vi "demo.vi"() -> ()   [LabVIEW 2012]
uses:
  <vilib>/Utility/miscctls.llb/LVPositionTypeDef.ctl
  SubVIs/typedef/User_Data_Cluster.ctl
  SubVIs/typedef/User Accounts.ctl
  type def/nodos.ctl
  type def/Hyde&Show.ctl
panel:
  out "INT \nRead":u16[](array[numeric])
  out "REAL \nRead":sgl[](array[numeric])
  out "BOOL \nRead":bool
  out "Cluster":T1
  in  "Video 2":bool
  in  "User-data cluster":T2
  out "Position":T4
  out "WS":picture
  out "Box":picture
  out "?":errorcluster
  in  "Admin Options":u16(ring)=1 items=["None", "1/ New User", "2/ Read&Modify Users", "3/ Read Log"]
  in  "Video":bool
  in  "?":bool
  in  "?":T5(tab)
  out "back ground":picture
  in  "error in (no error)":errorcluster
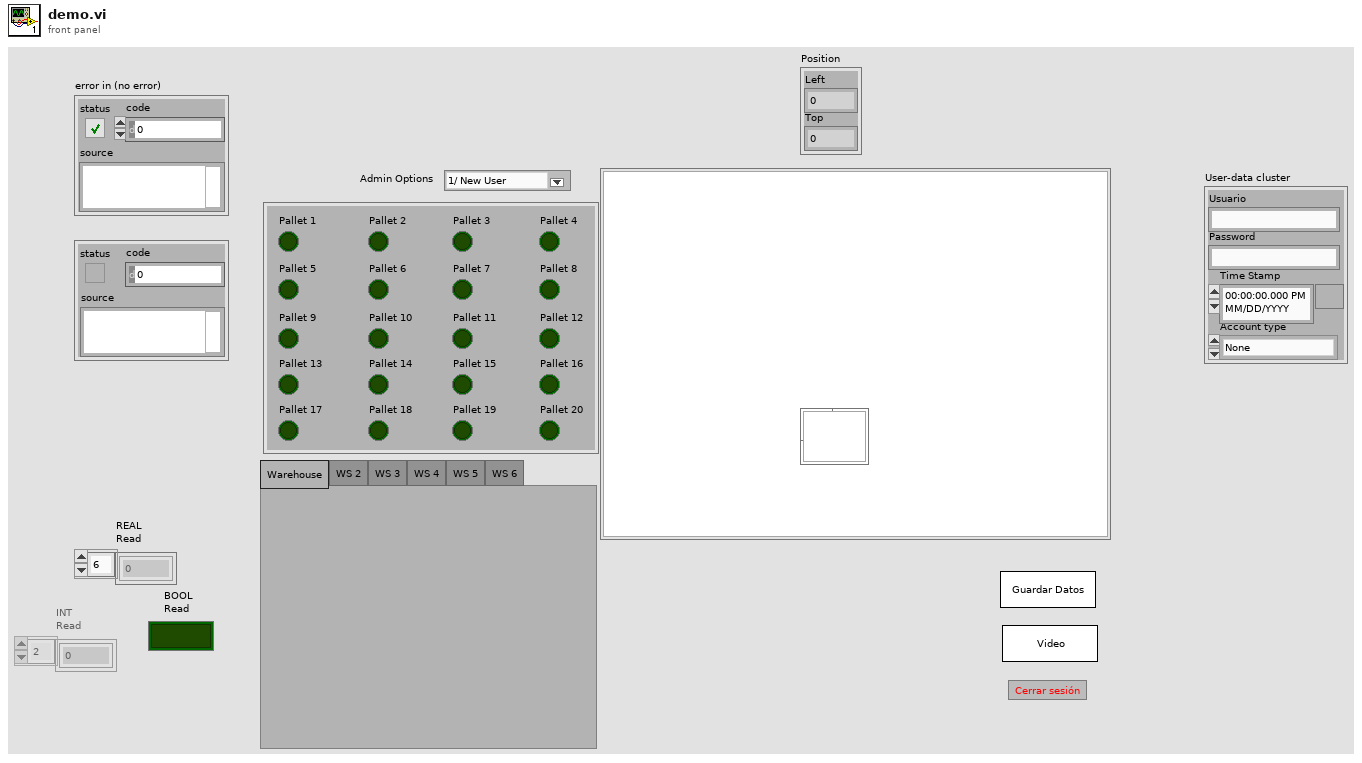
[diagram p1: front panel]
types:
  T1 = cluster{"Pallet 1":bool, "Pallet 2":bool, "Pallet 3":bool, "Pallet 4":bool, "Pallet 5":bool, "Pallet 6":bool, "Pallet 7":bool, "Pallet 8":bool, "Pallet 9":bool, "Pallet 10":bool, "Pallet 11":bool, "Pallet 12":bool, "Pallet 13":bool, "Pallet 14":bool, "Pallet 15":bool, "Pallet 16":bool, "Pallet 17":bool, "Pallet 18":bool, "Pallet 19":bool, "Pallet 20":bool}
  T2 = typedef "User_Data_Cluster.ctl" = cluster{"Usuario":string, "Password":string, "Account type":T3, "Time Stamp":timestamp}
  T3 = typedef "User Accounts.ctl" = enum16{"None", "User", "Admin"}
  T4 = typedef "LVPositionTypeDef.ctl" = cluster{"Left":i32, "Top":i32}
  T5 = enum32{"Warehouse", "WS 2", "WS 3", "WS 4", "WS 5", "WS 6"}
  T6 = cluster{"TCP Connection":refnum<k5>, "Session":u8[], "EtherNet/IP Device Address":string}
  T7 = typedef "nodos.ctl" = enum16{"Default", "Login", "Create", "Running", "Cluse User", "Close Conections", "End"}
  T8 = typedef "Hyde&Show.ctl" = enum8{"Enabled", "Disabled", "Disabled and Grayed Out", "Hide"}
  T9 = typedef "imagedata.ctl" = cluster{"image type":i32, "image depth":i32, "image":u8[], "mask":u8[], "colors":u32[], "Rectangle":cluster{"left":i16, "top":i16, "right":i16, "bottom":i16}}
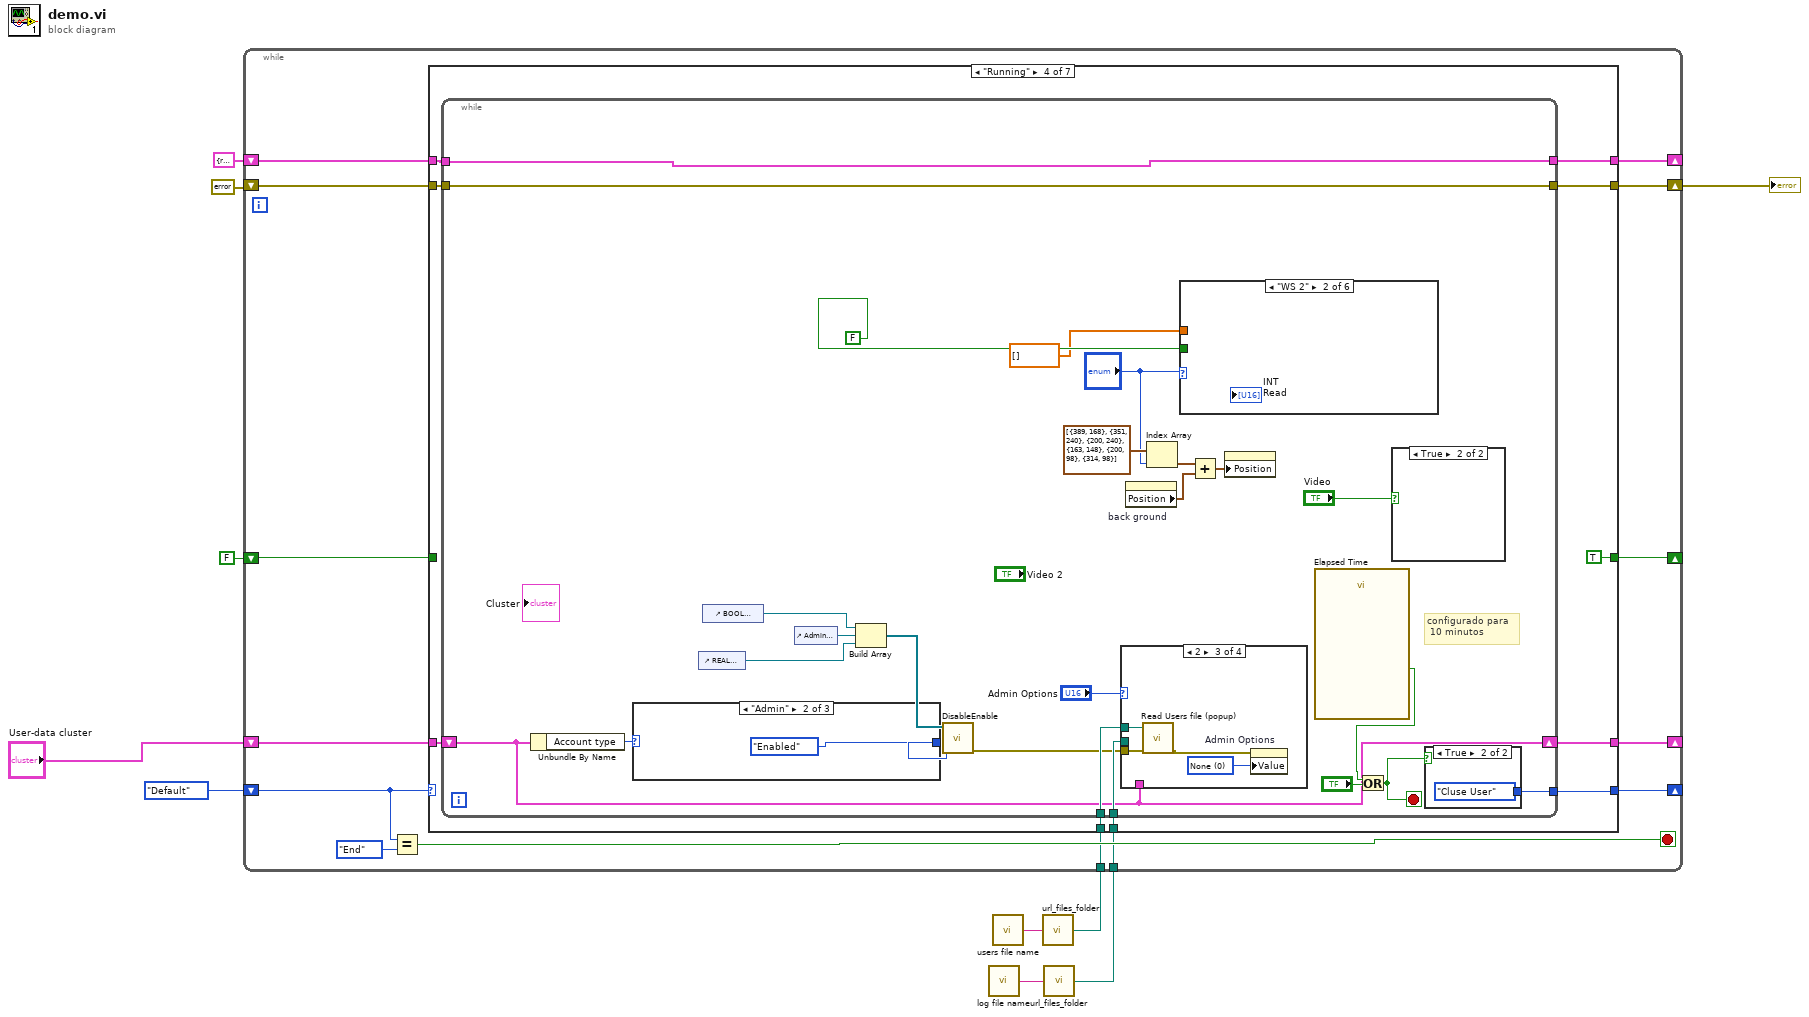
[diagram p0: block diagram]
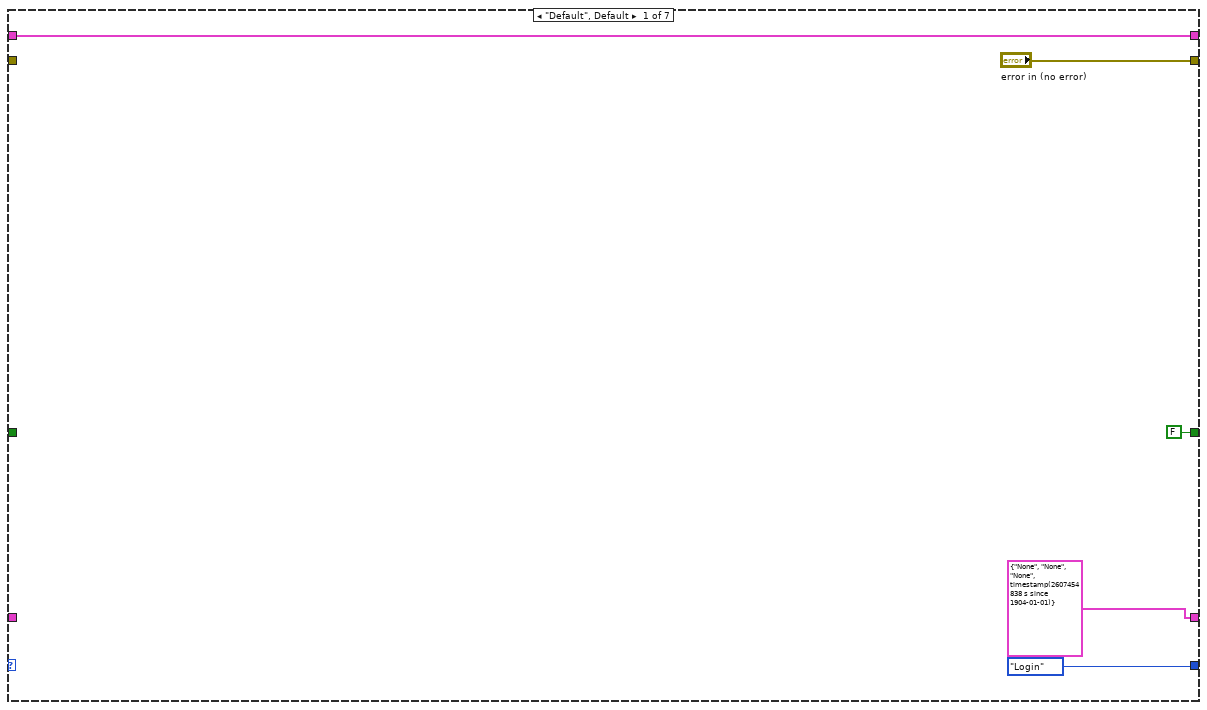
[diagram p2: hidden frame]
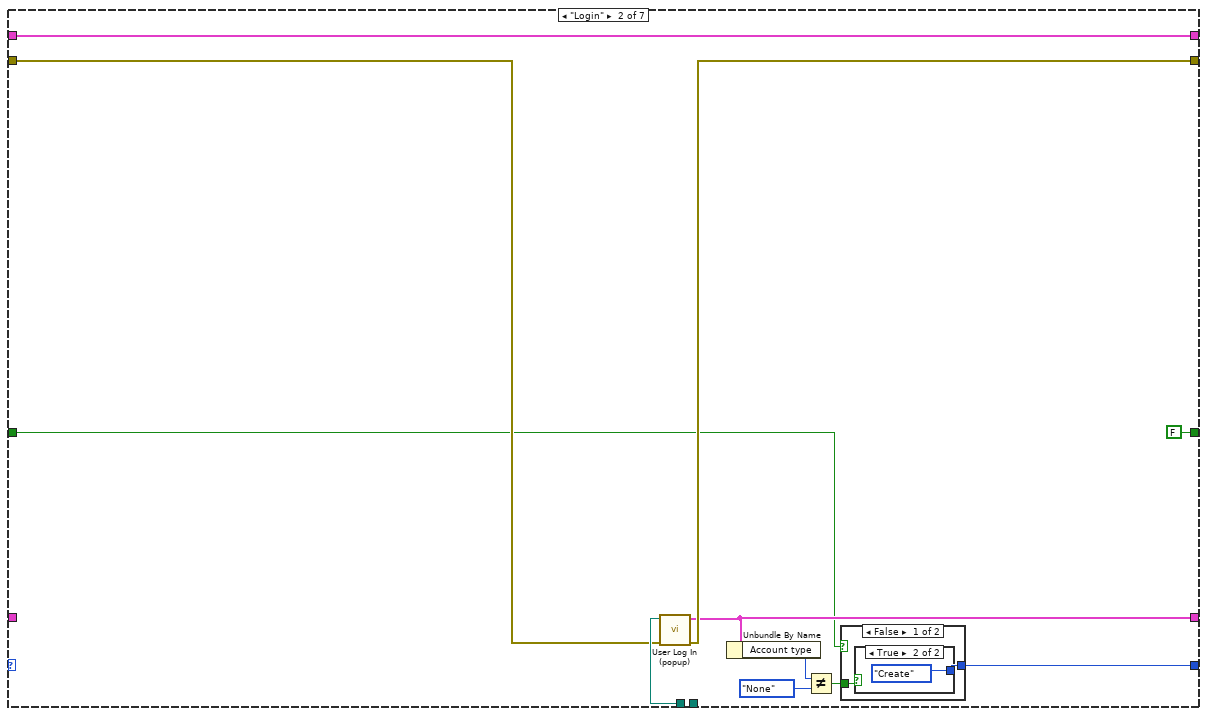
[diagram p3: hidden frame]
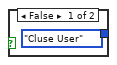
[diagram p4: hidden frame]
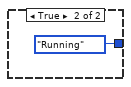
[diagram p5: hidden frame]
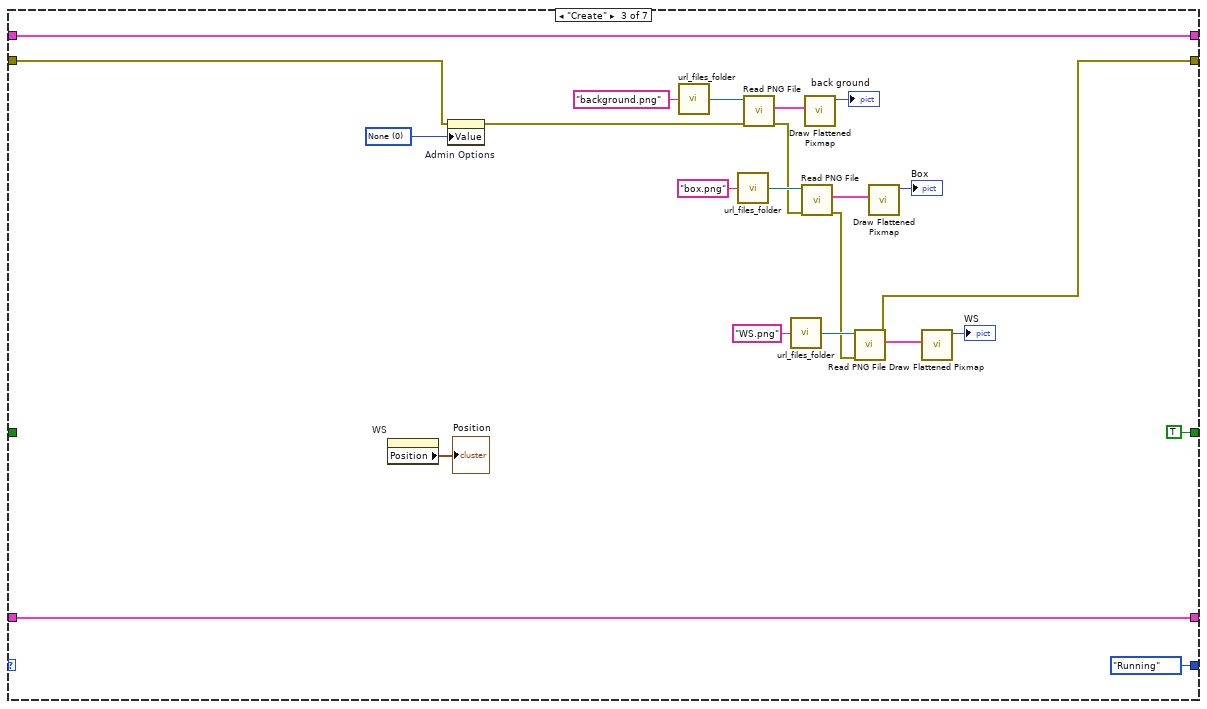
[diagram p6: hidden frame]
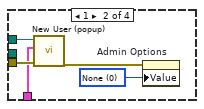
[diagram p8: hidden frame]
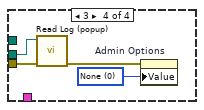
[diagram p9: hidden frame]
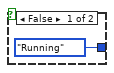
[diagram p10: hidden frame]
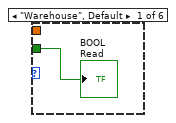
[diagram p12: hidden frame]
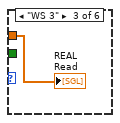
[diagram p13: hidden frame]
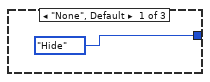
[diagram p17: hidden frame]
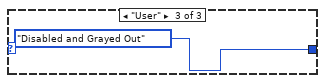
[diagram p18: hidden frame]
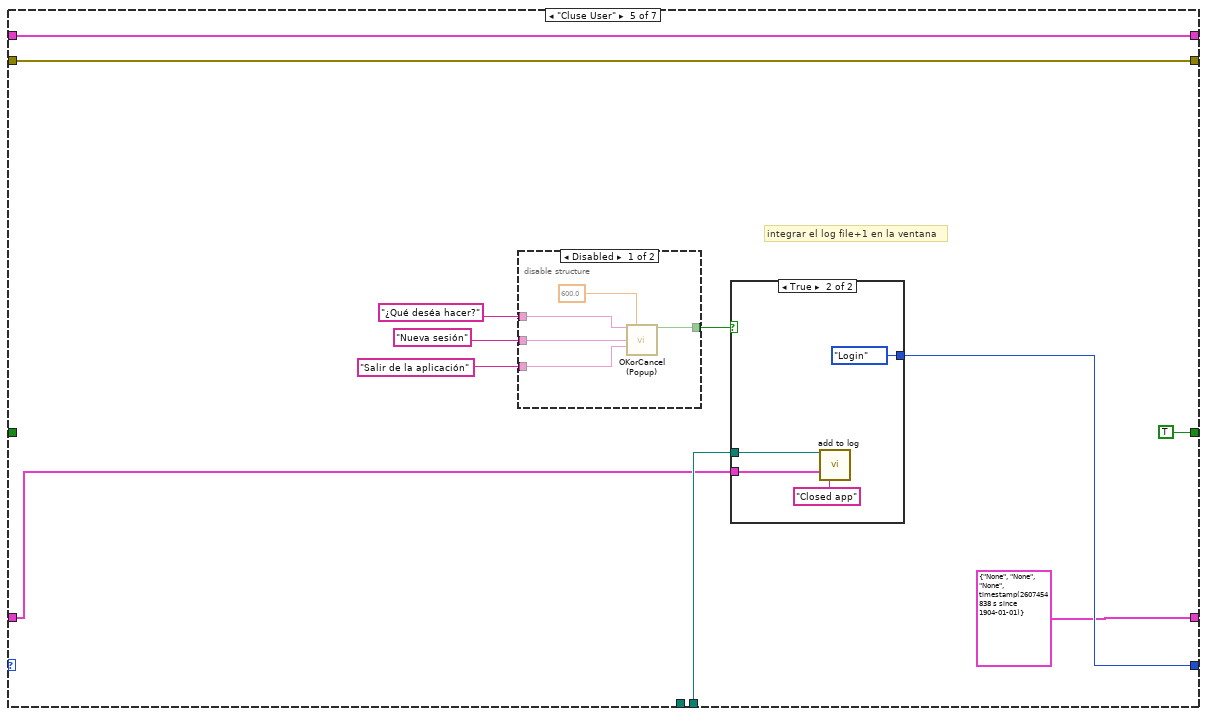
[diagram p19: hidden frame]
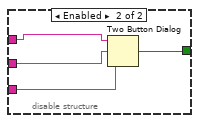
[diagram p20: hidden frame]
diagram:
  n1 = call "log file name.vi"() -> ("file name"=w4:string)  [unwired: 15 in]
  n2 = call "users file name.vi"() -> ("file name"=w6:string)  [unwired: 15 in]
  n3 = call "url_files_folder.vi"("file name"=w6) -> ("Path"=w5:path)  [unwired: 14 in]
  n4 = call "url_files_folder.vi"("file name"=w4) -> ("Path"=w3:path)  [unwired: 14 in]
  n5 = while {
    shift-right: [w23] -> _
    shift-left: nodos."Default" -> [w24]
    shift-right: [w16] -> w7
    shift-left: errorcluster {"status"=FALSE, "code"=0, "source"=""} ("error out") -> [w22]
    shift-right: [w19] -> _
    shift-left: "User-data cluster" -> [w17]
    shift-right: [w15] -> _
    shift-left: T6 {"TCP Connection"=refnum, "Session"=[], "EtherNet/IP Device Address"=""} ("Connection Cluster") -> [w18]
    tunnel: w5 -> [w14]
    tunnel: w3 -> [w13]
    shift-right: [w12] -> _
    shift-left: FALSE -> [w11]
    stop <- w20 stop-if-true
    n6 = Equal?(x=w24, y=nodos."End") -> (x = y?=w20:bool)
    n7 = case shown="\"Running\"" w24 {
      tunnel: [nodos."Login" w38 nodos."Running" w70 w134 nodos."End" nodos."End"] -> w23
      tunnel: ["error in (no error)" w34 w50 w75 w124 w149 w156] -> w16
      tunnel: w22 -> [_ w35 w47 w78 w124 w149 w156]
      tunnel: [T2 {"Usuario"="None", "Password"="None", "Account type"=enum."None", "Time Stamp"=timestamp(2607454838.413 s since 1904-01-01)} ("User-data cluster 2") w32 w64 w71 T2 {"Usuario"="None", "Password"="None", "Account type"=enum."None", "Time Stamp"=timestamp(2607454838.413 s since 1904-01-01)} ("User-data cluster 2") w152 T2 {"Usuario"="None", "Password"="None", "Account type"=enum."None", "Time Stamp"=timestamp(2607454838.413 s since 1904-01-01)} ("User-data cluster 2")] -> w19
      tunnel: w18 -> [w27 w36 w46 w77 w125 w150 w157]
      tunnel: w17 -> [_ _ w64 w74 w131 w152 _]
      tunnel: [w27 w36 w46 w76 w125 w150 w157] -> w15
      tunnel: w14 -> [_ w37 _ w72 _ _ _]
      tunnel: w13 -> [_ _ _ w73 w133 _ _]
      tunnel: [FALSE FALSE TRUE TRUE TRUE FALSE FALSE] -> w12
      tunnel: w11 -> [_ w30 _ _ _ _ _]
      frame "Default", Default {
      }
      frame "Login" {
        n8 = call "User Log In (popup).vi"("error in (no error)"=w35, 11:w37) -> ("error out"=w34:errorcluster, "User-data cluster Out"=w32:T2)  [unwired: 8 in]
        n9 = Unbundle By Name(w32) -> ("Account type"=w33:T3)
        n10 = Not Equal?(x=w33, y=User_Accounts."None") -> (x != y?=w40:bool)
        n11 = case shown="False" w30 {
          tunnel: w40 -> [w42 _]
          tunnel: [w41 nodos."Running"] -> w38
          frame False {
            n12 = case shown="True" w42 {
              tunnel: [nodos."Cluse User" nodos."Create"] -> w41
              frame False {
              }
              frame True {
              }
            }
          }
          frame True {
          }
        }
      }
      frame "Create" {
        w65 = u16 0 items=["None", "1/ View Users", "2/ Read Log", "3/ Modify Users", "4/ New User"] ("Admin Options")
        n13 = property on="WS" class="Pict"() -> ("Position"=→"Position":T4)  [unwired: 2 in, 2 out]
        n14 = property on="Admin Options" class="Ring (strict)"(error in=w47, "Value"=w65) -> (error out=w58:errorcluster)  [unwired: 1 in, 1 out]
        n15 = call "url_files_folder.vi"("file name"="background.png") -> ("Path"=w59:path)  [unwired: 14 in]
        n16 = call "url_files_folder.vi"("file name"="box.png") -> ("Path"=w60:path)  [unwired: 14 in]
        n17 = call <vilib>:"Read PNG File.vi"("error in (no error)"=w58, "path to PNG file"=w59) -> ("error out"=w57:errorcluster, "image data"=w68:T9)  [unwired: 7 in, 1 out]
        n18 = call "url_files_folder.vi"("file name"="WS.png") -> ("Path"=w53:path)  [unwired: 14 in]
        n19 = call <vilib>:"Read PNG File.vi"("error in (no error)"=w57, "path to PNG file"=w60) -> ("error out"=w51:errorcluster, "image data"=w66:T9)  [unwired: 7 in, 1 out]
        n20 = call <vilib>:"Draw Flattened Pixmap.vi"("image data"=w68) -> ("new picture"=→"back ground":picture)  [unwired: 8 in]
        n21 = call <vilib>:"Read PNG File.vi"("error in (no error)"=w51, "path to PNG file"=w53) -> ("error out"=w50:errorcluster, "image data"=w55:T9)  [unwired: 7 in, 1 out]
        n22 = call <vilib>:"Draw Flattened Pixmap.vi"("image data"=w66) -> ("new picture"=→"Box":picture)  [unwired: 8 in]
        n23 = call <vilib>:"Draw Flattened Pixmap.vi"("image data"=w55) -> ("new picture"=→"WS":picture)  [unwired: 8 in]
      }
      frame "Running" {
        n24 = while {
          tunnel: w78 -> [w81]
          tunnel: w77 -> [w82]
          tunnel: [w82] -> w76
          tunnel: [w81] -> w75
          shift-right: [w84] -> w71
          shift-left: w74 -> [w84]
          tunnel: w73 -> [w95]
          tunnel: w72 -> [w91]
          tunnel: [w94] -> w70
          stop <- w85 stop-if-true
          # "configurado para\n 10 minutos"
          n25 = Unbundle By Name(w84) -> ("Account type"=w88:T3)
          n26 = case shown="\"Admin\"" w88 {
            tunnel: [Hyde&Show."Hide" ("Action 2") Hyde&Show."Enabled" ("Action 2") Hyde&Show."Disabled and Grayed Out" ("Action 2")] -> w92
            frame "None", Default {
            }
            frame "Admin" {
            }
            frame "User" {
            }
          }
          n27 = control-ref of="REAL \nRead"() -> (w103:refnum<vi>)
          n28 = control-ref of="BOOL \nRead"() -> (w102:refnum<vi>)
          n29 = control-ref of="Admin Options"() -> (w101:refnum<vi>)
          n30 = Build Array(w102, w101, w103) -> (w93:refnum<vi>[])
          n31 = call "DisableEnable.vi"("Action 2"=w92, "Array of Control References"=w93) -> ("error out"=w90:errorcluster)  [unwired: 9 in]
          n32 = case shown="2" "Admin Options" {
            tunnel: w95 -> [_ _ _ w115]
            tunnel: w91 -> [_ w107 w111 _]
            tunnel: w90 -> [_ w105 w110 w113]
            tunnel: w84 -> [_ w104 _ _]
            frame 0, Default {
            }
            frame 1 {
              w108 = u16 0 items=["None", "1/ View Users", "2/ Read Log", "3/ Modify Users", "4/ New User"] ("Admin Options")
              n33 = call "New User (popup).vi"("error in (no error)"=w105, "User-data cluster"=w104, "file path (use dialog)"=w107) -> ("error out"=w106:errorcluster)  [unwired: 8 in]
              n34 = property on="Admin Options" class="Ring (strict)"(error in=w106, "Value"=w108) -> ()  [unwired: 1 in, 2 out]
            }
            frame 2 {
              w112 = u16 0 items=["None", "1/ View Users", "2/ Read Log", "3/ Modify Users", "4/ New User"] ("Admin Options")
              n35 = call "Read Users file (popup).vi"("file path (use dialog)"=w111, "error in (no error)"=w110) -> ("error out"=w109:errorcluster)  [unwired: 13 in]
              n36 = property on="Admin Options" class="Ring (strict)"(error in=w109, "Value"=w112) -> ()  [unwired: 1 in, 2 out]
            }
            frame 3 {
              w116 = u16 0 items=["None", "1/ View Users", "2/ Read Log", "3/ Modify Users", "4/ New User"] ("Admin Options")
              n37 = call "Read Log (popup).vi"("error in (no error)"=w113, "file path (use dialog)"=w115) -> ("error out"=w114:errorcluster)  [unwired: 9 in]
              n38 = property on="Admin Options" class="Ring (strict)"(error in=w114, "Value"=w116) -> ()  [unwired: 1 in, 2 out]
            }
          }
          n39 = property on="back ground" class="Pict"() -> ("Position"=w97:T4)  [unwired: 2 in, 2 out]
          n40 = Index Array(array=T4[] [{"Left"=389, "Top"=168}, {"Left"=351, "Top"=240}, {"Left"=200, "Top"=240}, {"Left"=163, "Top"=148}, {"Left"=200, "Top"=98}, {"Left"=314, "Top"=98}] ("Array"), index="?") -> (element=w98:T4)
          n41 = case shown="\"WS 2\"" "?" {
            tunnel: FALSE ("BOOL") -> [w119 _ _ _ _ _]
            tunnel: sgl[] [] ("REAL Array") -> [_ _ w120 _ _ _]
            frame "Warehouse", Default {
              "BOOL \nRead" <- w119
            }
            frame "WS 2" {
            }
            frame "WS 3" {
              "REAL \nRead" <- w120
            }
            frame "WS 4" {
            }
            frame "WS 5" {
            }
            frame "WS 6" {
            }
          }
          n42 = Add(x=w98, y=w97) -> (x+y=w83:T4)
          n43 = property on="Box" class="Pict"("Position"=w83) -> ()  [unwired: 2 in, 2 out]
          n44 = call "Elapsed Time"() -> ("Time has Elapsed"=w86:bool)  [unwired: 12 in, 7 out]
          n45 = Or(x=w86, y="?") -> (x .or. y?=w85:bool)
          n46 = case shown="True" "Video" {
            frame False {
            }
            frame True {
            }
          }
          n47 = case shown="True" w85 {
            tunnel: [nodos."Running" nodos."Cluse User"] -> w94
            frame False {
            }
            frame True {
            }
          }
        }
      }
      frame "Cluse User" {
        # "integrar el log file+1 en la ventana"
        n48 = disable-structure shown="Disabled" {
          disable-tunnel: [w139 w143] -> w130
          disable-tunnel: "¿Qué deséa hacer?" ("message") -> [w137 w142]
          disable-tunnel: "Nueva sesión" ("T button name (\"OK\")") -> [w136 w141]
          disable-tunnel: "Salir de la aplicación" ("F button name (\"Cancel\")") -> [w135 w140]
          frame Disabled {
            n49 = call "OKorCancel (Popup).vi"("message"=w137, "Seconds before TimeOut"=600.0, "T button name (\"OK\")"=w136, "F button name (\"Cancel\")"=w135) -> ("T button?"=w139:bool)  [unwired: 9 in, 2 out]
          }
          frame Enabled {
            n50 = Two Button Dialog(message=w142, 1:w140, 2:w141) -> (T button?=w143:bool)
          }
        }
        n51 = case shown="True" w130 {
          tunnel: [nodos."Close Conections" nodos."Login"] -> w134
          tunnel: w133 -> [_ w147]
          tunnel: w131 -> [_ w145]
          frame False {
          }
          frame True {
            n52 = call "add to log.vi"("Path"=w147, "User-data cluster"=w145, "Data"="Closed app") -> ()  [unwired: 13 in]
          }
        }
      }
      frame "Close Conections" {
      }
      frame "End" {
      }
    }
  }
  "?" <- w7
